vi "Finish.vi"   [LabVIEW 2012]
doc: "This VI is called just before exiting. It is expected to close I/O refnum, save collected data, etc."
uses:
  Robot Global Data.vi
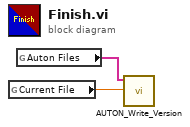
[diagram p0: block diagram]
diagram:
  n1 = global read "Robot Global Data.vi" "Current File"() -> (w2:dbl)
  n2 = global read "Robot Global Data.vi" "Auton Files"() -> (w1:string[])
  n3 = call "AUTON_Write_Version.vi"("Current File"=w2, "Auton Files"=w1) -> ()  [unwired: 10 in]
